vi "CM-Write Configuration.vi"(0 "Connection File Path":path, 2 "Section":string, 7 "Endpoints":T1[](array[typedef]), 11 "error in (no error)":errorcluster) -> (4 "Path Out":path, 15 "error out":errorcluster)   [LabVIEW 2020]
uses:
  Typedefs/CM-Endpoint.ctl
  <vilib>/Utility/config.llb/Write Key (String).vi
  <vilib>/Utility/config.llb/NI_LVConfig.lvlib
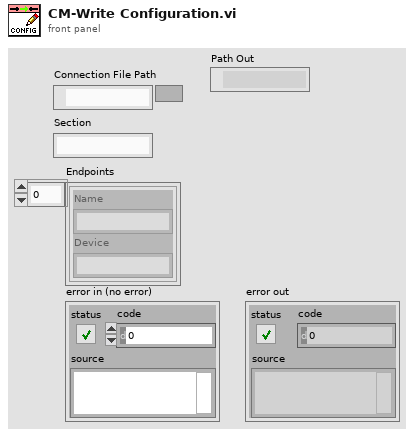
[diagram p1: front panel]
types:
  T1 = typedef "CM-Endpoint.ctl" = cluster{"Name":string, "Device":string}
  T2 = typedef "NI_LVConfig.lvlib/Config Data RefNum.ctl" = refnum<k1>
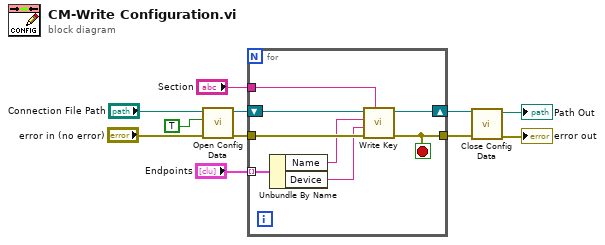
[diagram p0: block diagram]
diagram:
  n1 = call <vilib>:"Open Config Data.vi"("error in (no error)"="error in (no error)", "create file if necessary (T)"=TRUE, "configuration file path"="Connection File Path") -> ("error out"=w8:errorcluster, "refnum"=w10:T2)  [unwired: 6 in, 1 out]
  n2 = for {
    tunnel: "Section" -> [w18]
    tunnel: w8 -> [w17]
    tunnel: [w16] -> w7
    shift-right: [w15] -> w6
    shift-left: w10 -> [w19]
    tunnel: "Endpoints" -> [w14] mode=indexing
    stop <- w16 stop-if-true
    n3 = Unbundle By Name(w14) -> ("Name"=w13:string, "Device"=w12:string)
    n4 = call-poly <vilib>:"Write Key.vi"("section"=w18, "error in (no error)"=w17, "value"=w12, "key"=w13, "refnum"=w19) -> ("error out"=w16:errorcluster, "refnum out"=w15:T2)  [unwired: 4 in, 1 out]
  }
  n5 = call <vilib>:"Close Config Data.vi"("error in (no error)"=w7, "refnum"=w6) -> ("error out"=→"error out":errorcluster, "file path"=→"Path Out":path)  [unwired: 8 in]
